vi "Control Panel Actuators.vi"(10 "Wheel":dbl(slide) scale=-1.0..1.0, 11 "Arm":dbl(slide) scale=-1.0..1.0) -> (3 "Control Panel Motors":T1)   [LabVIEW 2019]
uses:
  Control Panel Motors.ctl
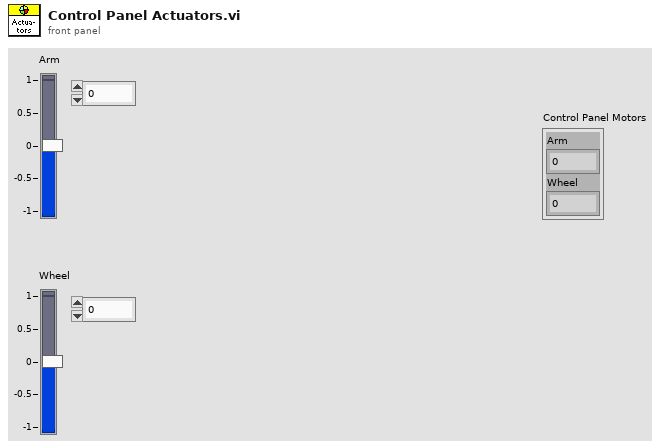
[diagram p1: front panel]
types:
  T1 = typedef "Control Panel Motors.ctl" = cluster{"Arm":dbl, "Wheel":dbl}
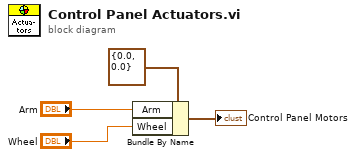
[diagram p0: block diagram]
diagram:
  n1 = Bundle By Name(cluster=T1 {"Arm"=0.0, "Wheel"=0.0} ("Color Wheel Motors"), "Arm"="Arm", "Wheel"="Wheel") -> (→"Control Panel Motors":T1)
